vi "SelectMenu3.vi"(6 "Click Type":T1, 7 "Id":string, 8 "Point":T4, 9 "Item Index":u32, 10 "XRef":refnum<vi>, 11 "State In":T2) -> (0 "Reply":string[](array[string]), 3 "State Out":T2)   [LabVIEW 2012, in "CRefScripting.lvlib" / "CRef Label Node.xnode"]
doc: "This ability VI is called after the user selects an item from a portion of the menu defined during BuildMenu. Click Type is the type of click that led to the building of the menu whose selection is being handled by this VI. ItemIndex is the index of the element in the array used when you specified the popup menu. Id is the id you associated with the item in BuildMenu3. Point is the location where the user clicked to build the menu relative to the top-left corner of the XNode. You can display a dialog in response to a user selection if you wish. Use Reply to inform LabVIEW of any actions it needs to take.\n\nDefault behavior: None.\n\nThis ability provides UI and OS messages are handled.\n\nSee also: BuildMenu3"
uses:
  CRef Label Node.xnode
  State.ctl
  Core/Master Types.ctl
  <vilib>/XNodeSupport/XNodePoint.ctl
  <vilib>/XNodeSupport/XNodeInt.ctl
  <vilib>/XNodeSupport/XNodeClickTypes.ctl
  <vilib>/XNodeSupport/NI_XNodeSupport.lvlib
  CRef.lvlib
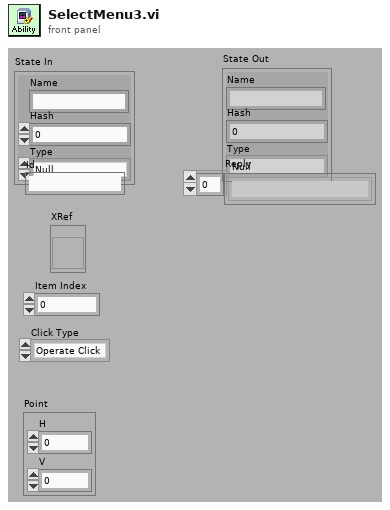
[diagram p1: front panel]
types:
  T1 = typedef "NI_XNodeSupport.lvlib/XNodeClickTypes.ctl" = enum32{"Operate Click", "Popup Click"}
  T2 = typedef "CRefScripting.lvlib/CRef Label Node.xnode/State.ctl" = cluster{"Name":string, "Hash":u32, "Type":T3}
  T3 = typedef "CRef.lvlib/Master Types.ctl" = enum8{"Null", "Boolean", "U8", "I8", "U16", "I16", "U32", "I32", "U64", "I64", "Single", "Double", "Extended", "CSG", "CDB", "CXT", "Boolean(Def)", "U8(Def)", "I8(Def)", "U16(Def)", "I16(Def)", "U32(Def)", "I32(Def)", "Reserved Def", "Reserved Def1", "Single(Def)", "Double(Def)", "Reserved Def2", "Reserved Def3", "Reserved Def4", "Reserved Def5", "Unsigned(Def)", "Signed(Def)", "Real(Def)", "Reserved Def6", "Numeric(Def)", "String"}
  T4 = typedef "NI_XNodeSupport.lvlib/XNodePoint.ctl" = cluster{"H":T5, "V":T5}
  T5 = typedef "NI_XNodeSupport.lvlib/XNodeInt.ctl" = i32
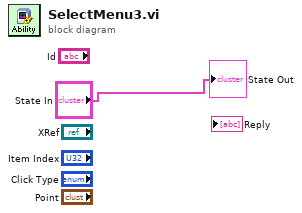
[diagram p0: block diagram]
diagram:
  "State Out" <- "State In"
